vi "Add.vi"(8 "error in (no error)":errorcluster, 11 "Status Actor in":refnum<class "Status Actor.lvclass">) -> (0 "error out":errorcluster, 3 "Status Actor out":refnum<class "Status Actor.lvclass">)   [LabVIEW 2019, in "Status Actor.lvlib" / "Status Actor.lvclass"]
uses:
  Status Actor.lvclass
  Status Actor.lvclass/Status Actor.ctl
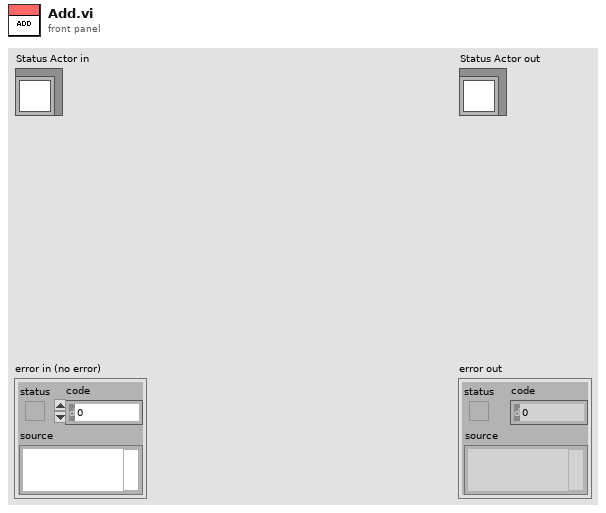
[diagram p1: front panel]
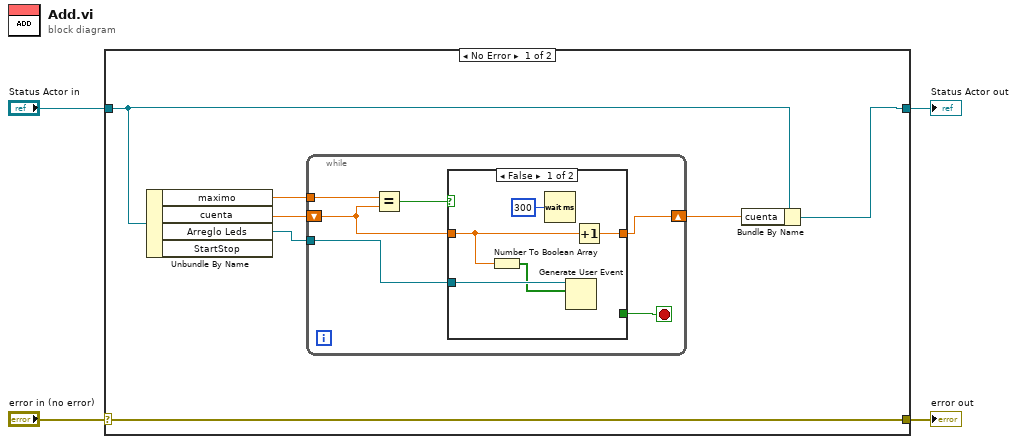
[diagram p0: block diagram]
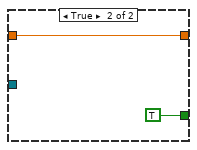
[diagram p2: hidden frame]
diagram:
  n1 = case shown="No Error" "error in (no error)" {
    selector: "error in (no error)" -> [w11 w26]
    tunnel: [w11 w26] -> w3
    tunnel: [w9 w25] -> w1
    tunnel: "Status Actor in" -> [w10 w25]
    frame No Error {
      n2 = Unbundle By Name(w10) -> ("maximo"=w6:dbl, "cuenta"=w8:dbl, "Arreglo Leds"=w5:refnum<user-event>)  [unwired: 1 out]
      n3 = while {
        tunnel: w6 -> [w14]
        tunnel: w5 -> [w13]
        shift-right: [w15] -> w7
        shift-left: w8 -> [w16]
        stop <- w12 stop-if-true
        n4 = Equal?(x=w14, y=w16) -> (x = y?=w17:bool)
        n5 = case shown="False" w17 {
          tunnel: w16 -> [w20 w24]
          tunnel: [w22 w24] -> w15
          tunnel: w13 -> [w21 _]
          tunnel: [_ TRUE] -> w12
          frame False {
            n6 = Number To Boolean Array(number=w20) -> (Boolean array=w19:bool[])
            n7 = Wait (ms)(milliseconds to wait=u32 300) -> ()  [unwired: 1 out]
            n8 = Generate User Event(user event=w21, event data cluster=w19) -> ()  [unwired: 2 in, 2 out]
            n9 = Increment(x=w20) -> (x+1=w22:dbl)
          }
          frame True {
          }
        }
      }
      n10 = Bundle By Name(cluster=w10, "cuenta"=w7) -> (w9:refnum<class "Status Actor.lvclass">)
    }
    frame Error {
    }
  }
  "error out" <- w3
  "Status Actor out" <- w1
